vi "GetStringMatch.vi"(8 "error in (no error)":errorcluster, 9 "Reject Regex":string, 10 "Match Regex":string, 11 "String":string[](array[string])) -> (0 "error out":errorcluster, 3 "Matching string":string)   [LabVIEW 2019, in "LINXx.lvlib"]
uses:
  <vilib>/regexp/Match Regular Expression.xnode
  LINXx.lvlib
panel:
  out "Match?":bool
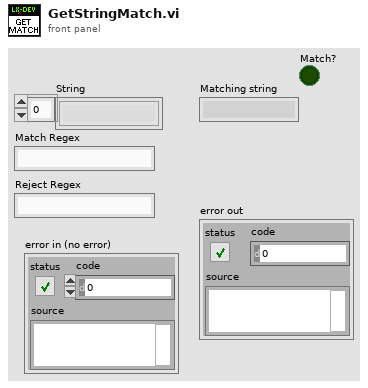
[diagram p1: front panel]
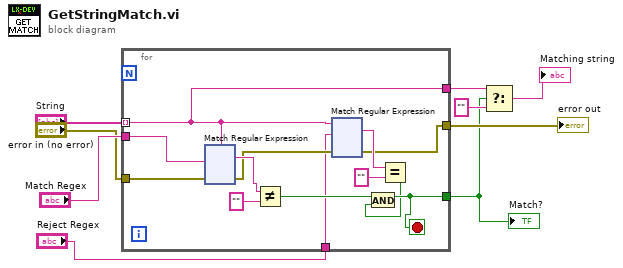
[diagram p0: block diagram]
diagram:
  n1 = for {
    tunnel: "String" -> [w12] mode=indexing
    tunnel: "error in (no error)" -> [w20]
    tunnel: [w14] -> w4
    tunnel: [w12] -> w6
    tunnel: [w10] -> w8
    tunnel: "Match Regex" -> [w18]
    tunnel: "Reject Regex" -> [w11]
    stop <- w14 stop-if-true
    n2 = xnode "Match Regular Expression"("input string"=w12, "regular expression"=w18, "error in"=w20) -> ("whole match"=w21:string, "error out"=w17:errorcluster)  [unwired: 3 in, 3 out]
    n3 = Not Equal?(x=w21, y="") -> (x != y?=w19:bool)
    n4 = xnode "Match Regular Expression"("input string"=w12, "regular expression"=w11, "error in"=w17) -> ("whole match"=w15:string, "error out"=w10:errorcluster)  [unwired: 3 in, 3 out]
    n5 = Equal?(x=w15, y="") -> (x = y?=w13:bool)
    n6 = And(x=w19, y=w13) -> (x .and. y?=w14:bool)
  }
  "error out" <- w8
  "Match?" <- w4
  n7 = Select(t=w6, s=w4, f="") -> (s? t:f=→"Matching string":string)
